vi "Create directory.vi"(8 "error in (no error)":errorcluster, 11 "Identifier 1":string) -> (0 "error out":errorcluster, 3 "created path":path)   [LabVIEW 2016]
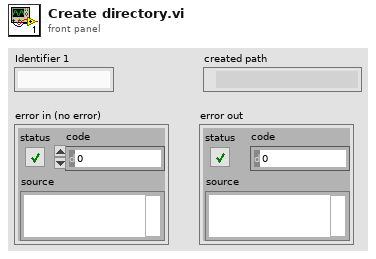
[diagram p1: front panel]
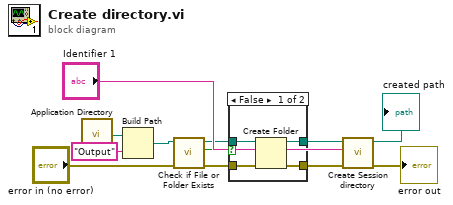
[diagram p0: block diagram]
diagram:
  n1 = call <vilib>:"Application Directory.vi"() -> ("Application Directory"=w3:path)
  n2 = Build Path(base path=w3, name or relative path="Output") -> (appended path=w5:path)
  n3 = call <vilib>:"Check if File or Folder Exists.vi"("error in (no error)"="error in (no error)", "path"=w5) -> ("error out"=w8:errorcluster, "file or folder exists?"=w7:bool, "dup path"=w10:path)  [unwired: 7 in]
  n4 = case shown="False" w7 {
    tunnel: w8 -> [w16 w18]
    tunnel: [w13 w18] -> w9
    tunnel: w10 -> [w15 w17]
    tunnel: [w14 w17] -> w11
    frame False {
      n5 = Create Folder(path (use dialog)=w15, error in=w16) -> (created path=w14:path, error out=w13:errorcluster)  [unwired: 1 in, 1 out]
    }
    frame True {
    }
  }
  n6 = call "Create Session directory.vi"("error in (no error)"=w9, "Identifier 1"="Identifier 1", "appended path"=w11) -> ("error out"=→"error out":errorcluster, "created path"=→"created path":path)  [unwired: 6 in, 1 out]
